vi "ex14-15.vi"() -> ()   [LabVIEW 2014]
uses:
  <vilib>/NXT/Subs/MotorOutput.ctl
  <vilib>/NXT/Dual Mode Library/Motors/MotorDistance_Single.vi
panel:
  out "X XOR Y-二進位陣列顯示":dbl[](array[numeric])
  out "X XOR Y":i32
  out "Y-二進位顯示":dbl[](array[numeric])
  in  "Y":dbl
  in  "X":dbl
  out "X-二進位顯示":dbl[](array[numeric])
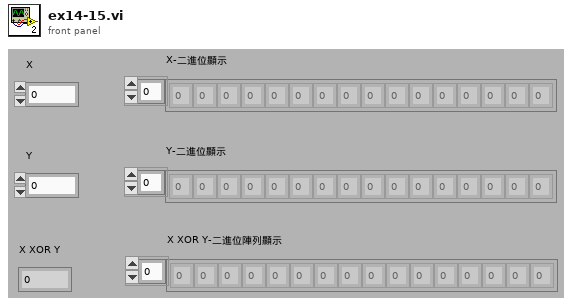
[diagram p1: front panel]
types:
  T1 = typedef "MotorOutput.ctl" = u8
  T2 = typedef "LVHSConnector.ctl" = refnum<class "BrickReference.lvclass">
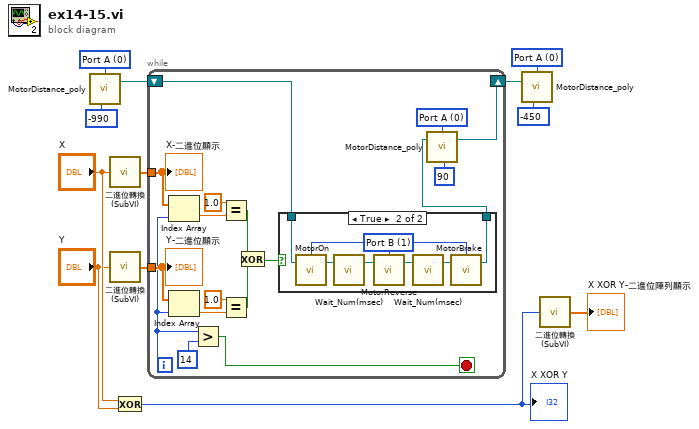
[diagram p0: block diagram]
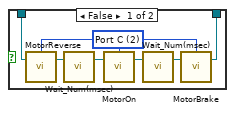
[diagram p2: hidden frame]
diagram:
  w7 = T1 0 items=["Port A", "Port B", "Port C", "All Ports"] ("Output Port (All Ports)")
  w9 = T1 0 items=["Port A", "Port B", "Port C", "All Ports"] ("Output Port (All Ports)")
  n1 = call-poly <vilib>:"MotorDistance_poly.vi"("Angle of Rotation (360)"=-990 ("Distance (100)"), "Output Port (All Ports)"=w9) -> ("NXT/EV3"=w8:T2)  [unwired: 2 in]
  n2 = call "二進位轉換 (SubVI).vi"("十進位"="X") -> ("二進位"=w12:dbl[])
  n3 = call "二進位轉換 (SubVI).vi"("十進位"="Y") -> ("二進位"=w11:dbl[])
  n4 = Exclusive Or(1:"Y", 2:"X") -> (0:w1:i32)
  "X XOR Y" <- w1
  n5 = while {
    tunnel: w12 -> [w29]
    tunnel: w11 -> [w28]
    shift-right: [w13] -> w5
    shift-left: w8 -> [w17]
    i -> [w27]
    stop <- w25 stop-if-true
    w15 = T1 0 items=["Port A", "Port B", "Port C", "All Ports"] ("Output Port (All Ports)")
    n6 = Index Array(array=w29, index=w27) -> (element=w21:dbl)
    n7 = Index Array(array=w28, index=w27) -> (element=w22:dbl)
    n8 = Greater?(x=w27, y=14) -> (0:w25:bool)
    n9 = Equal?(x=1.0, y=w21) -> (x = y?=w19:bool)
    n10 = Equal?(x=1.0, y=w22) -> (x = y?=w20:bool)
    n11 = Exclusive Or(1:w20, 2:w19) -> (0:w18:bool)
    n12 = case shown="True" w18 {
      tunnel: w17 -> [w31 w38]
      tunnel: [w30 w37] -> w14
      frame False {
        w36 = T1 2 items=["Port A", "Port B", "Port C", "All Ports"] ("Output Port (All Ports)")
        n13 = call <vilib>:"MotorReverse.vi"("NXT/EV3"=w31, "Output Port (All Ports)"=w36) -> ("NXT/EV3"=w32:T2)  [unwired: 2 in]
        n14 = call <vilib>:"Wait_Num(msec).vi"("NXT/EV3"=w32) -> ("NXT/EV3"=w33:T2)  [unwired: 3 in]
        n15 = call <vilib>:"MotorOn.vi"("NXT/EV3"=w33, "Output Port (All Ports)"=w36) -> ("NXT/EV3"=w34:T2)  [unwired: 2 in]
        n16 = call <vilib>:"Wait_Num(msec).vi"("NXT/EV3"=w34) -> ("NXT/EV3"=w35:T2)  [unwired: 3 in]
        n17 = call <vilib>:"MotorBrake.vi"("NXT/EV3"=w35, "Port (All Ports)"=w36) -> ("NXT/EV3"=w30:T2)  [unwired: 2 in]
      }
      frame True {
        w39 = T1 1 items=["Port A", "Port B", "Port C", "All Ports"] ("Output Port (All Ports)")
        n18 = call <vilib>:"MotorOn.vi"("NXT/EV3"=w38, "Output Port (All Ports)"=w39) -> ("NXT/EV3"=w43:T2)  [unwired: 2 in]
        n19 = call <vilib>:"Wait_Num(msec).vi"("NXT/EV3"=w43) -> ("NXT/EV3"=w42:T2)  [unwired: 3 in]
        n20 = call <vilib>:"MotorReverse.vi"("NXT/EV3"=w42, "Output Port (All Ports)"=w39) -> ("NXT/EV3"=w41:T2)  [unwired: 2 in]
        n21 = call <vilib>:"Wait_Num(msec).vi"("NXT/EV3"=w41) -> ("NXT/EV3"=w40:T2)  [unwired: 3 in]
        n22 = call <vilib>:"MotorBrake.vi"("NXT/EV3"=w40, "Port (All Ports)"=w39) -> ("NXT/EV3"=w37:T2)  [unwired: 2 in]
      }
    }
    n23 = call-poly <vilib>:"MotorDistance_poly.vi"("Angle of Rotation (360)"=90 ("Distance (100)"), "NXT/EV3"=w14, "Output Port (All Ports)"=w15) -> ("NXT/EV3"=w13:T2)  [unwired: 1 in]
    "X-二進位顯示" <- w29
    "Y-二進位顯示" <- w28
  }
  n24 = call-poly <vilib>:"MotorDistance_poly.vi"("Angle of Rotation (360)"=-450 ("Distance (100)"), "NXT/EV3"=w5, "Output Port (All Ports)"=w7) -> ()  [unwired: 1 in, 1 out]
  n25 = call "二進位轉換 (SubVI).vi"("十進位"=w1) -> ("二進位"=→"X XOR Y-二進位陣列顯示":dbl[])
